vi "Controller.vi"() -> ()   [LabVIEW 2020]
uses:
  C:/GEECS/Developers Version/source/Device Drivers/KinesisCube/Thorlabs.MotionControl.Controls.dll
  Thorlabs.MotionControl.Controls.dll
  C:/GEECS/Developers Version/source/Device Drivers/KinesisCube/Thorlabs.MotionControl.KCube.PiezoCLI.dll
  Thorlabs.MotionControl.KCube.PiezoCLI.dll
panel:
  in  "enable 150 V\nDefault is 75 V":bool
  in  "enable":bool
  in  "delayTime":i32
  in  "state":i32(ring) items=["Disconnected", "Connecting", "PreConnecting", "Connected"]
  in  "voltageSource 2":i32(ring) items=["SoftwareOnly", "ExternalSignal", "Potentiometer"]
  out "CreateDevice":bool
  in  "volts":dbl
  out "GetOutputVoltage":sgl
  in  "stop":bool
  in  "SerialNumber":string="29250543"
  in  "KCubePiezoControl":refnum<k24>(container)
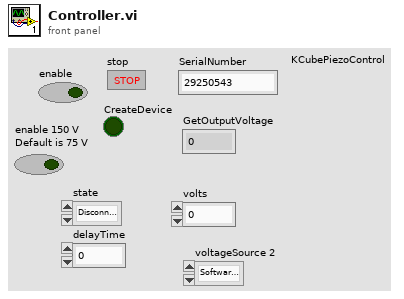
[diagram p1: front panel]
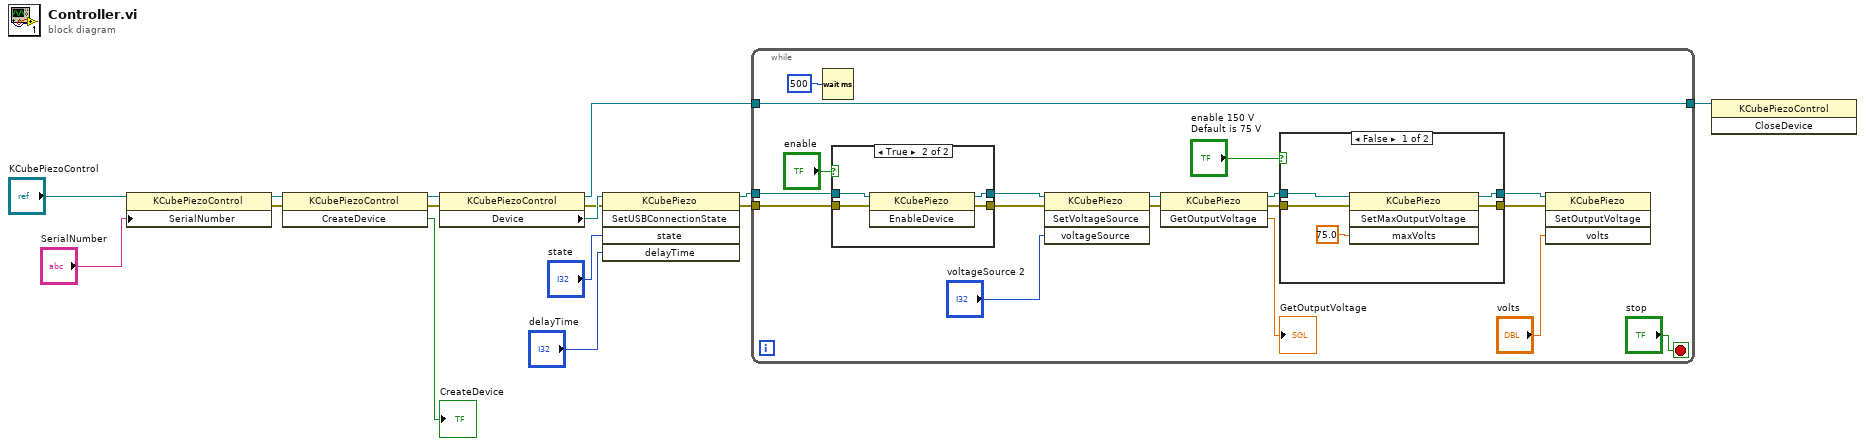
[diagram p0: block diagram]
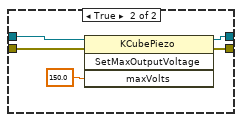
[diagram p2: hidden frame]
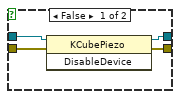
[diagram p3: hidden frame]
diagram:
  n1 = property class="KCubePiezoControl"(reference="KCubePiezoControl", "SerialNumber"="SerialNumber") -> (reference out=w13:refnum<k24>, error out=w11:errorcluster)  [unwired: 1 in]
  n2 = invoke class="KCubePiezoControl" method="CreateDevice"(reference=w13, error in=w11) -> (reference out=w12:refnum<k24>, error out=w10:errorcluster, "CreateDevice"=→"CreateDevice":bool)  [unwired: 1 in]
  n3 = property class="KCubePiezoControl"(reference=w12, error in=w10) -> (reference out=w9:refnum<k24>, error out=w2:errorcluster, "Device"=w4:refnum<k24>)
  n4 = invoke class="KCubePiezo" method="SetUSBConnectionState"(reference=w4, error in=w2, "state"="state", "delayTime"="delayTime") -> (reference out=w3:refnum<k24>, error out=w1:errorcluster)  [unwired: 1 in, 3 out]
  n5 = while {
    tunnel: w9 -> [w30]
    tunnel: [w30] -> w8
    tunnel: w3 -> [w26]
    tunnel: w1 -> [w25]
    stop <- "stop" stop-if-true
    n6 = Wait (ms)(milliseconds to wait=u32 500) -> ()  [unwired: 1 out]
    n7 = case shown="True" "enable" {
      tunnel: w26 -> [w46 w51]
      tunnel: w25 -> [w47 w50]
      tunnel: [w45 w49] -> w24
      tunnel: [w44 w48] -> w23
      frame False {
        n8 = invoke class="KCubePiezo" method="DisableDevice"(reference=w46, error in=w47) -> (reference out=w45:refnum<k24>, error out=w44:errorcluster)  [unwired: 1 in, 1 out]
      }
      frame True {
        n9 = invoke class="KCubePiezo" method="EnableDevice"(reference=w51, error in=w50) -> (reference out=w49:refnum<k24>, error out=w48:errorcluster)  [unwired: 1 in, 1 out]
      }
    }
    n10 = invoke class="KCubePiezo" method="SetVoltageSource"(reference=w24, error in=w23, "voltageSource"="voltageSource 2") -> (reference out=w28:refnum<k24>, error out=w27:errorcluster)  [unwired: 1 in, 2 out]
    n11 = invoke class="KCubePiezo" method="GetOutputVoltage"(reference=w28, error in=w27) -> (reference out=w19:refnum<k24>, error out=w17:errorcluster, "GetOutputVoltage"=→"GetOutputVoltage":dbl)  [unwired: 1 in]
    n12 = case shown="False" "enable 150 V\nDefault is 75 V" {
      tunnel: w19 -> [w37 w42]
      tunnel: [w36 w39] -> w18
      tunnel: w17 -> [w35 w41]
      tunnel: [w34 w40] -> w16
      frame False {
        n13 = invoke class="KCubePiezo" method="SetMaxOutputVoltage"(reference=w37, error in=w35, "maxVolts"=75.0) -> (reference out=w36:refnum<k24>, error out=w34:errorcluster)  [unwired: 1 in, 2 out]
      }
      frame True {
        n14 = invoke class="KCubePiezo" method="SetMaxOutputVoltage"(reference=w42, error in=w41, "maxVolts"=150.0) -> (reference out=w39:refnum<k24>, error out=w40:errorcluster)  [unwired: 1 in, 2 out]
      }
    }
    n15 = invoke class="KCubePiezo" method="SetOutputVoltage"(reference=w18, error in=w16, "volts"="volts") -> ()  [unwired: 1 in, 4 out]
  }
  n16 = invoke class="KCubePiezoControl" method="CloseDevice"(reference=w8) -> ()  [unwired: 2 in, 3 out]
